vi "ge_GetGlblString.vi"(4 "Value":variant, 5 "ge_DAQManDefinitions":T1, 6 "Label.Text":string, 7 "MeasType":T2, 8 "error in":errorcluster, 9 "Row":i32, 10 "Header":string, 11 "Device":string) -> (0 "error out":errorcluster, 2 "Cell Contents":T3[](array[typedef]))   [LabVIEW 2018]
uses:
  Custom Ctls Table/ge_CellContents.ctl
  <vilib>/Utility/miscctls.llb/LVPoint32TypeDef.ctl
  Custom Ctrls/ge_MeasType.ctl
  Common/Controls/DAQMan Definitions.ctl
  Custom Ctls Table/ge_ColType.ctl
  Common/Controls/HeaderNames.ctl
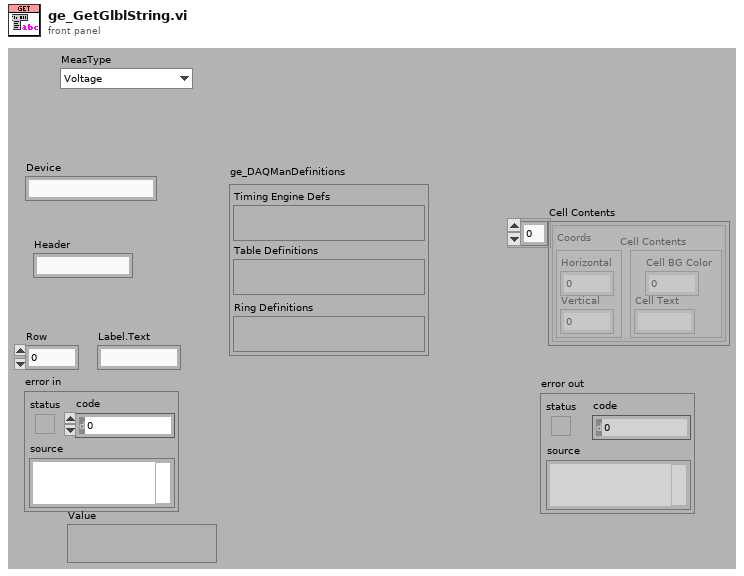
[diagram p1: front panel]
types:
  T1 = typedef "DAQMan Definitions.ctl" = cluster{"Timing Engine Defs":variant, "Table Definitions":variant, "Ring Definitions":variant}
  T2 = typedef "ge_MeasType.ctl" = enum16{"Voltage", "Frequency", "Tachometer", "Dynamic", "Thermocouple", "RTD", "Strain", "Current", "Resistance"}
  T3 = typedef "ge_CellContents.ctl" = cluster{"Cell Contents":cluster{"Cell Text":string, "Cell BG Color":u32}, "Coords":T4}
  T4 = typedef "LVPoint32TypeDef.ctl" = cluster{"Horizontal":i32, "Vertical":i32}
  T5 = typedef "ge_GlblCtrls.ctl" = enum16{"Str0", "Bool0", "Bool1", "Int0", "Ring0", "Ring1", "Ring2", "Ring3", "Dbl0", "Dbl1", "Dbl2", "Dbl3", "Cal0", "Cal1", "Cal2", "None"}
  T6 = typedef "HeaderNames.ctl" = enum16{"Channel", "Device", "Spacer", "Description", "MB", "Range", "Terminal", "Coupling", "Thresh (V)", "Pulse/Rev", "Slope", "Min EU", "Min RPM", "mV/EU", "Iex", "Temp Units", "Type", "CJC Src", "CJC Val", "Ro", "Wire Cfg", "Strain Mode", "Vex", "Bridge Type", "GF", "Gauge Res", "Poisson", "Lead Res", "Init Strain", "GAF", "Scale", "Offset", "Unit (EU)", "dB?", "dB Ref", "Cal Mag", "Cal Units", "Max Temp", "Min Temp", "Max Strain", "Min Strain"}
  T7 = typedef "ge_ColType.ctl" = enum16{"Volts", "Amps", "Ohms", "TermCfg", "WireCfg", "Coup", "Slope", "Iex", "CalUnits", "ThrmUnits", "ThrmType", "CJCSrc", "BrdgType", "Strn Mode", "RTDType"}
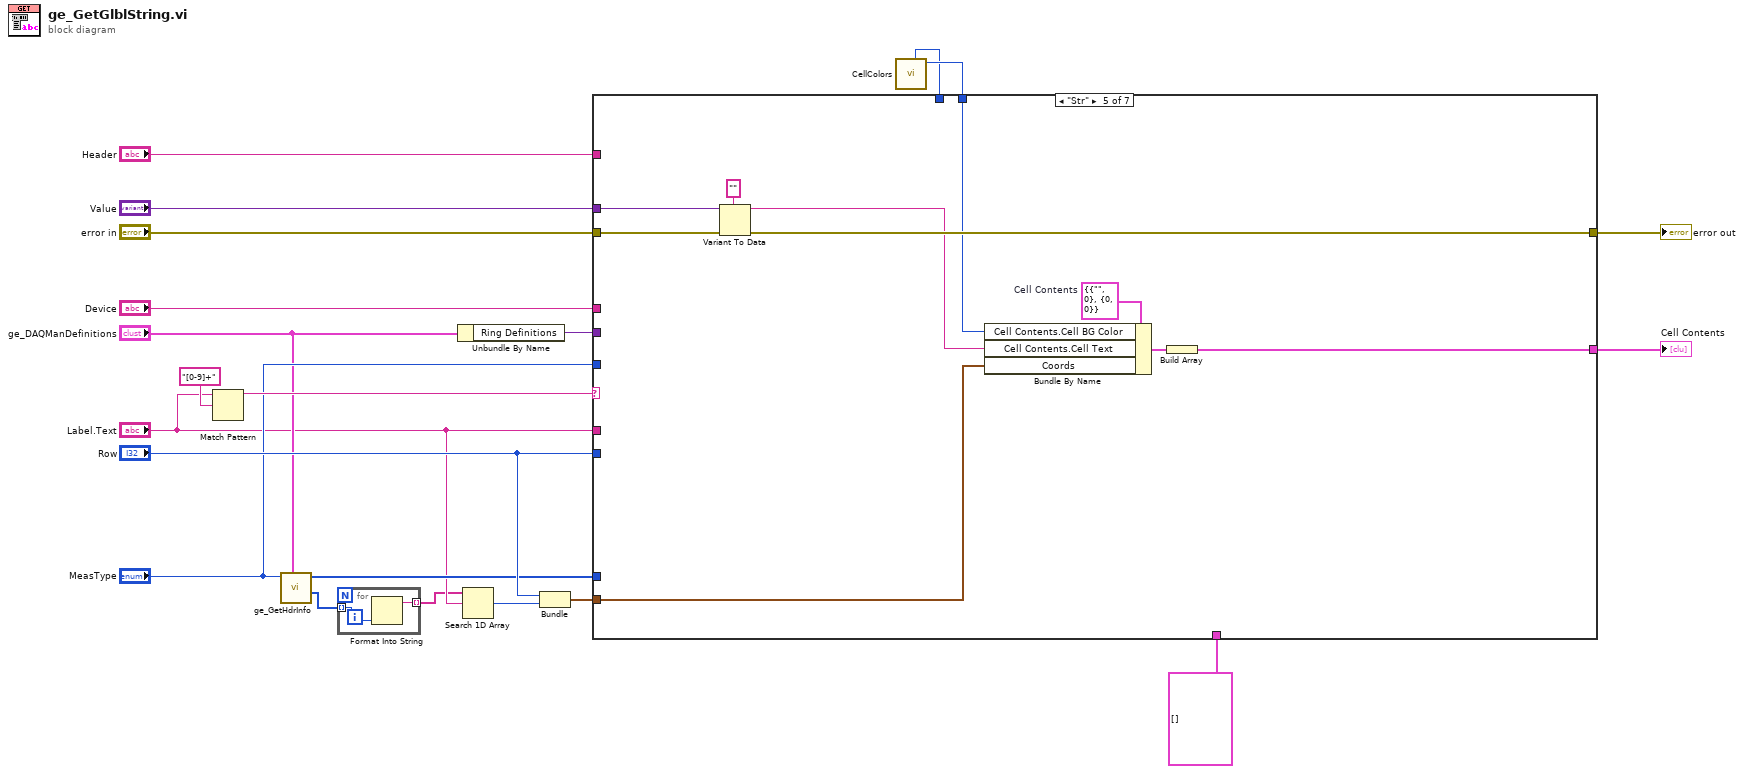
[diagram p0: block diagram]
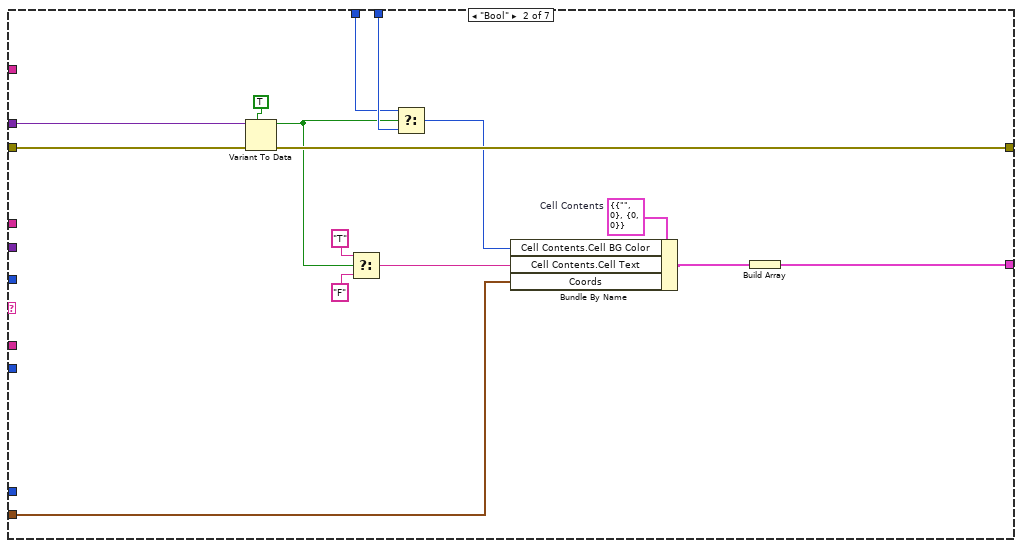
[diagram p3: hidden frame]
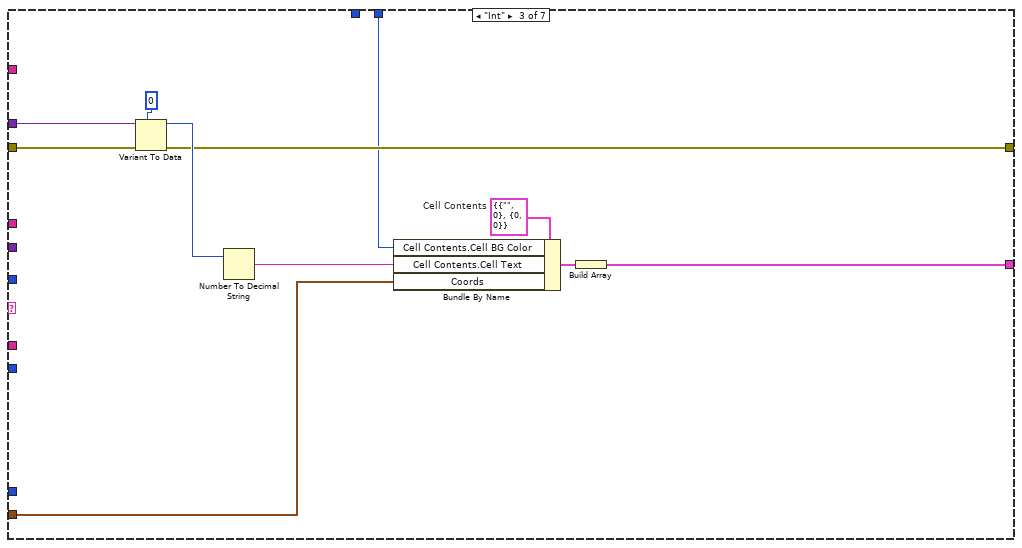
[diagram p4: hidden frame]
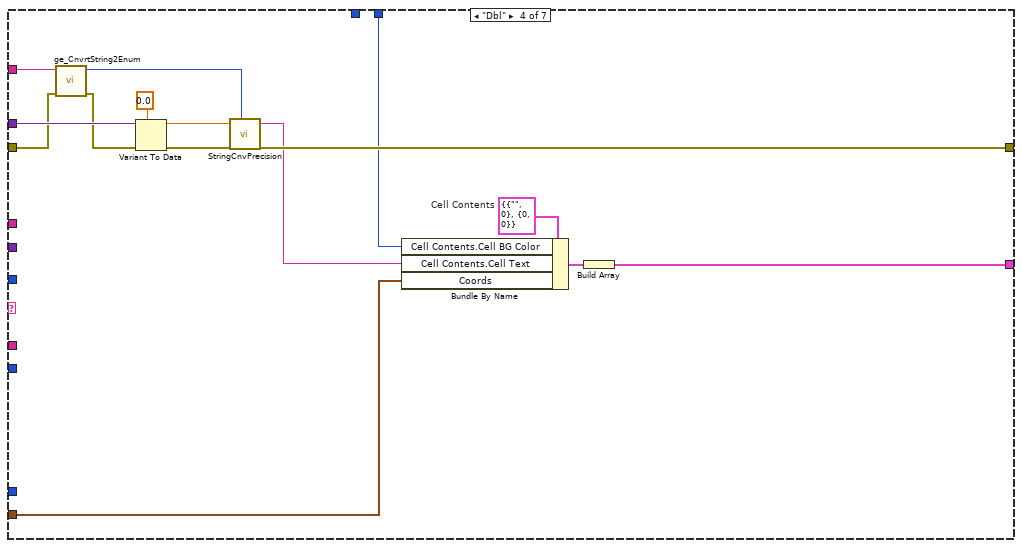
[diagram p5: hidden frame]
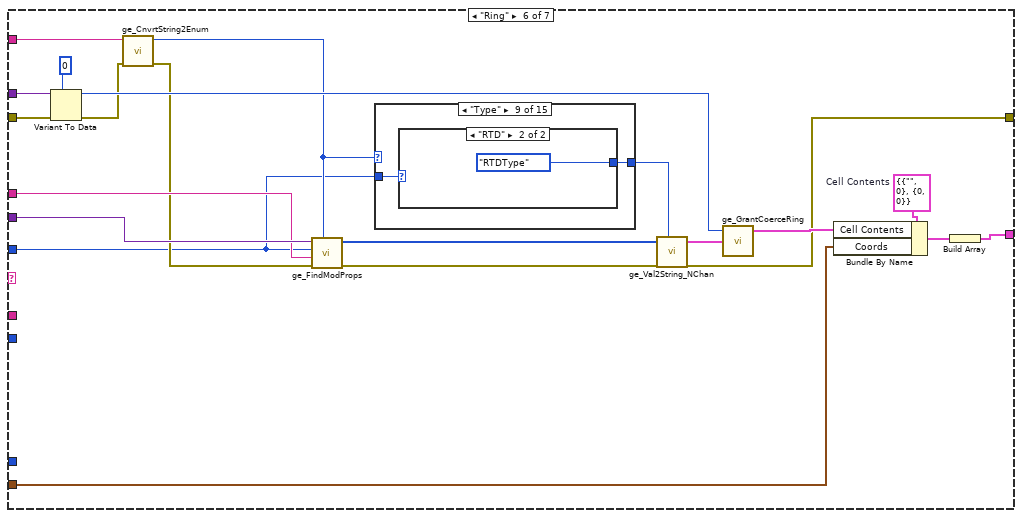
[diagram p6: hidden frame]
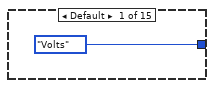
[diagram p7: hidden frame]
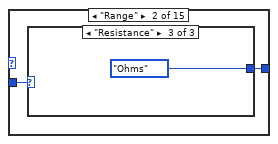
[diagram p8: hidden frame]
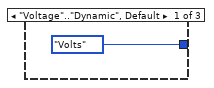
[diagram p9: hidden frame]
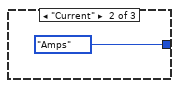
[diagram p10: hidden frame]
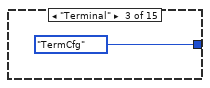
[diagram p11: hidden frame]
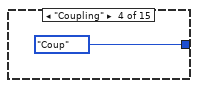
[diagram p12: hidden frame]
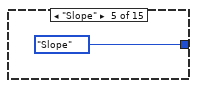
[diagram p13: hidden frame]
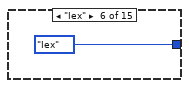
[diagram p14: hidden frame]
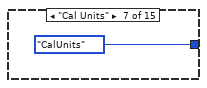
[diagram p15: hidden frame]
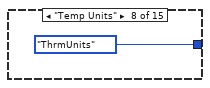
[diagram p16: hidden frame]
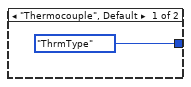
[diagram p17: hidden frame]
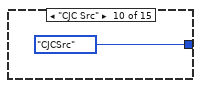
[diagram p18: hidden frame]
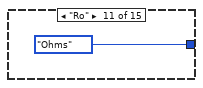
[diagram p19: hidden frame]
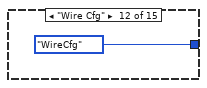
[diagram p20: hidden frame]
diagram:
  n1 = Match Pattern(string="Label.Text", regular expression="[0-9]+") -> (before substring=w13:string)  [unwired: 1 in, 3 out]
  n2 = call "ge_GetHdrInfo.vi"("ge_DAQManDefinitions"="ge_DAQManDefinitions", "MeasType"="MeasType") -> ("Glbl Ctrls"=w1:T5[], "Hdr Name"=w14:T6[])  [unwired: 7 in, 1 out]
  n3 = for {
    tunnel: w1 -> [w23] mode=indexing
    tunnel: [w22] -> w2 mode=indexing
    n4 = Format Into String(w23) -> (resulting string=w22:string)  [unwired: 3 in, 1 out]
  }
  n5 = Unbundle By Name("ge_DAQManDefinitions") -> ("Ring Definitions"=w5:variant)
  n6 = Search 1D Array(1D array=w2, element="Label.Text") -> (index of element=w7:i32)  [unwired: 1 in]
  n7 = Bundle("Row"="Row", "index of element"=w7) -> (w6:cluster{"Row":i32, "index of element":i32})  [unwired: 1 in]
  n8 = call "CellColors.vi"() -> ("Normal"=w17:u32, "True"=w16:u32)  [unwired: 8 in, 2 out]
  n9 = case shown="\"Str\"" w13 {
    tunnel: w5 -> [_ _ _ _ _ w83 _]
    tunnel: "Device" -> [_ _ _ _ _ w82 _]
    tunnel: "error in" -> [w25 w38 w49 w53 w75 w94 w131]
    tunnel: [w25 w37 w48 w65 w74 w84 w131] -> w20
    tunnel: [w24 w30 w45 w62 w68 w89 w129] -> w15
    tunnel: w17 -> [_ w40 w43 w61 w71 _ w130]
    tunnel: w16 -> [_ w39 _ _ _ _ _]
    tunnel: "Label.Text" -> [_ _ _ _ _ _ w121]
    tunnel: "Header" -> [_ _ _ w55 _ w79 _]
    tunnel: "Value" -> [_ w27 w42 w59 w67 w87 _]
    tunnel: w6 -> [_ w26 w41 w58 w66 w86 _]
    tunnel: T3[] [] -> [w24 _ _ _ _ _ _]
    tunnel: "MeasType" -> [_ _ _ _ _ w77 w122]
    tunnel: w14 -> [_ _ _ _ _ _ w126]
    tunnel: "Row" -> [_ _ _ _ _ _ w125]
    frame Default {
    }
    frame "Bool" {
      w32 = T3 {"Cell Contents"={"Cell Text"="", "Cell BG Color"=0}, "Coords"={"Horizontal"=0, "Vertical"=0}}  # Cell Contents
      n10 = Variant To Data(error in=w38, type=TRUE, Variant=w27) -> (data=w33:bool, error out=w37:errorcluster)
      n11 = Select(t="T" ("Default String"), s=w33, f="F" ("Default String")) -> (s? t:f=w29:string)
      n12 = Select(t=w39, s=w33, f=w40) -> (s? t:f=w28:u32)
      n13 = Bundle By Name(cluster=w32, "Cell Contents.Cell BG Color"=w28, "Cell Contents.Cell Text"=w29, "Coords"=w26) -> (w31:T3)
      n14 = Build Array(w31) -> (w30:T3[])
    }
    frame "Int" {
      w47 = T3 {"Cell Contents"={"Cell Text"="", "Cell BG Color"=0}, "Coords"={"Horizontal"=0, "Vertical"=0}}  # Cell Contents
      n15 = Variant To Data(error in=w49, type=u32 0, Variant=w42) -> (data=w50:u32, error out=w48:errorcluster)
      n16 = Number To Decimal String(number=w50) -> (decimal integer string=w44:string)  [unwired: 1 in]
      n17 = Bundle By Name(cluster=w47, "Cell Contents.Cell BG Color"=w43, "Cell Contents.Cell Text"=w44, "Coords"=w41) -> (w46:T3)
      n18 = Build Array(w46) -> (w45:T3[])
    }
    frame "Dbl" {
      w63 = T3 {"Cell Contents"={"Cell Text"="", "Cell BG Color"=0}, "Coords"={"Horizontal"=0, "Vertical"=0}}  # Cell Contents
      n19 = call "ge_CnvrtString2Enum.vi"("error in (no error)"=w53, "Enum String"=w55) -> ("error out"=w52:errorcluster, "Hdr Name"=w54:T6)  [unwired: 8 in]
      n20 = Variant To Data(error in=w52, type=0.0, Variant=w59) -> (data=w56:dbl, error out=w65:errorcluster)
      n21 = call "StringCnvPrecision.vi"("Number"=w56, "Header"=w54) -> ("Float String"=w57:string)  [unwired: 5 in]
      n22 = Bundle By Name(cluster=w63, "Cell Contents.Cell BG Color"=w61, "Cell Contents.Cell Text"=w57, "Coords"=w58) -> (w60:T3)
      n23 = Build Array(w60) -> (w62:T3[])
    }
    frame "Str" {
      w72 = T3 {"Cell Contents"={"Cell Text"="", "Cell BG Color"=0}, "Coords"={"Horizontal"=0, "Vertical"=0}}  # Cell Contents
      n24 = Variant To Data(error in=w75, type="", Variant=w67) -> (data=w70:string, error out=w74:errorcluster)
      n25 = Bundle By Name(cluster=w72, "Cell Contents.Cell BG Color"=w71, "Cell Contents.Cell Text"=w70, "Coords"=w66) -> (w69:T3)
      n26 = Build Array(w69) -> (w68:T3[])
    }
    frame "Ring" {
      w91 = T3 {"Cell Contents"={"Cell Text"="", "Cell BG Color"=0}, "Coords"={"Horizontal"=0, "Vertical"=0}}  # Cell Contents
      n27 = Variant To Data(error in=w94, type=u16 0 ("Glbl Iex"), Variant=w87) -> (data=w93:u16, error out=w80:errorcluster)
      n28 = call "ge_CnvrtString2Enum.vi"("error in (no error)"=w80, "Enum String"=w79) -> ("error out"=w81:errorcluster, "Hdr Name"=w78:T6)  [unwired: 8 in]
      n29 = call "ge_FindModProps.vi"("Hdr Name"=w78, "error in (no error)"=w81, "Device"=w82, "MeasType"=w77, "All Ring Support"=w83) -> ("error out"=w84:errorcluster, "Values"=w85:u16[])  [unwired: 5 in]
      n30 = case shown="\"Type\"" w78 {
        tunnel: [ge_ColType."Volts" ("ColType") w98 ge_ColType."TermCfg" ("ColType") ge_ColType."Coup" ("ColType") ge_ColType."Slope" ("ColType") ge_ColType."Iex" ("ColType") ge_ColType."CalUnits" ("ColType") ge_ColType."ThrmUnits" ("ColType") w108 ge_ColType."CJCSrc" ("ColType") ge_ColType."Ohms" ("ColType") ge_ColType."WireCfg" ("ColType") ge_ColType."Strn Mode" ("ColType") ge_ColType."Volts" ("ColType") ge_ColType."BrdgType" ("ColType")] -> w76
        tunnel: w77 -> [_ w97 _ _ _ _ _ _ w109 _ _ _ _ _ _]
        frame Default {
        }
        frame "Range" {
          n31 = case shown="\"Resistance\"" w97 {
            tunnel: [ge_ColType."Volts" ("ColType") ge_ColType."Amps" ("ColType") ge_ColType."Ohms" ("ColType")] -> w98
            frame "Voltage".."Dynamic", Default {
            }
            frame "Current" {
            }
            frame "Resistance" {
            }
          }
        }
        frame "Terminal" {
        }
        frame "Coupling" {
        }
        frame "Slope" {
        }
        frame "Iex" {
        }
        frame "Cal Units" {
        }
        frame "Temp Units" {
        }
        frame "Type" {
          n32 = case shown="\"RTD\"" w109 {
            tunnel: [ge_ColType."ThrmType" ("ColType") ge_ColType."RTDType" ("ColType")] -> w108
            frame "Thermocouple", Default {
            }
            frame "RTD" {
            }
          }
        }
        frame "CJC Src" {
        }
        frame "Ro" {
        }
        frame "Wire Cfg" {
        }
        frame "Strain Mode" {
        }
        frame "Vex" {
        }
        frame "Bridge Type" {
        }
      }
      n33 = call "ge_Val2String_NChan.vi"("Values"=w85, "ColType"=w76) -> ("String and Values"=w92:cluster{"String":string, "Value":u16}[])  [unwired: 5 in]
      n34 = call "ge_GrantCoerceRing.vi"("String and Values"=w92, "Requested Value"=w93) -> ("Cel Val and Color"=w88:cluster{"Value":string, "Color":u32})  [unwired: 3 in]
      n35 = Bundle By Name(cluster=w91, "Cell Contents"=w88, "Coords"=w86) -> (w90:T3)
      n36 = Build Array(w90) -> (w89:T3[])
    }
    frame "Cal" {
      n37 = case shown="\"Voltage\"" w122 {
        tunnel: HeaderNames."Channel" ("element") -> [w132 w134 _]
        tunnel: [w132 HeaderNames."Offset" ("element") HeaderNames."Init Strain" ("element")] -> w120
        tunnel: [w132 w134 HeaderNames."GAF" ("element")] -> w119
        frame Default {
        }
        frame "Voltage" {
        }
        frame "Strain" {
        }
      }
      n38 = Search 1D Array(1D array=w126, element=w120) -> (index of element=w128:i32)  [unwired: 1 in]
      n39 = Search 1D Array(1D array=w126, element=w119) -> (index of element=w127:i32)  [unwired: 1 in]
      n40 = Bundle("Row"=w125, "index of element"=w128) -> (w124:cluster{"Row":i32, "index of element":i32})  [unwired: 1 in]
      n41 = Bundle("Row"=w125, "index of element"=w127) -> (w123:cluster{"Row":i32, "index of element":i32})  [unwired: 1 in]
      n42 = case shown="\"Cal0\"" w121 {
        tunnel: [T3[] [] w143 w151] -> w129
        tunnel: w124 -> [_ w139 w150]
        tunnel: w130 -> [_ w140 w148]
        tunnel: w123 -> [_ _ w147]
        frame Default {
        }
        frame "Cal0" {
          w141 = T3 {"Cell Contents"={"Cell Text"="", "Cell BG Color"=0}, "Coords"={"Horizontal"=0, "Vertical"=0}}  # Cell Contents
          n43 = Bundle By Name(cluster=w141, "Cell Contents.Cell BG Color"=w140, "Cell Contents.Cell Text"="0.00" ("Cell Color/Text.Cell Text"), "Coords"=w139) -> (w138:T3)
          n44 = Build Array(w138) -> (w143:T3[])
        }
        frame "Cal1" {
          w149 = T3 {"Cell Contents"={"Cell Text"="", "Cell BG Color"=0}, "Coords"={"Horizontal"=0, "Vertical"=0}}  # Cell Contents
          n45 = Bundle By Name(cluster=w149, "Cell Contents.Cell BG Color"=w148, "Cell Contents.Cell Text"="0.00" ("Cell Color/Text.Cell Text"), "Coords"=w150) -> (w152:T3)
          n46 = Bundle By Name(cluster=w149, "Cell Contents.Cell BG Color"=w148, "Cell Contents.Cell Text"="1.00" ("Cell Color/Text.Cell Text"), "Coords"=w147) -> (w144:T3)
          n47 = Build Array(w152, w144) -> (w151:T3[])
        }
      }
    }
  }
  "error out" <- w20
  "Cell Contents" <- w15
